vi "q1 x1_x2_2.vi"(8 "x2":dbl, 11 "x1":dbl) -> (2 "(x1-x2)^2":dbl)   [LabVIEW 2025]
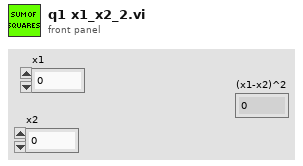
[diagram p1: front panel]
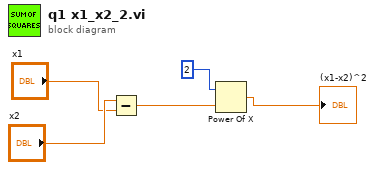
[diagram p0: block diagram]
diagram:
  n1 = Subtract(x="x2", y="x1") -> (x-y=w3:dbl)
  n2 = Power Of X(1:w3, 2:2) -> (0:→"(x1-x2)^2":dbl)
